vi "Init Msg Output.vi"() -> (2 "Msg Output":refnum<class "Msg Output.lvclass">)   [LabVIEW 2020, in "jettl.lvlib" / "Stop jettl Msg.lvlib" / "Stop Msg Output.lvlib"]
uses:
  Stop Msg Output.lvlib
  Msg Output/Msg Output.lvclass
  Stop Msg Output/Stop Msg Output.lvclass
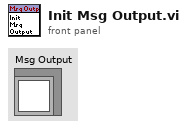
[diagram p1: front panel]
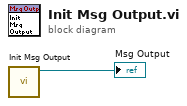
[diagram p0: block diagram]
diagram:
  n1 = call "Init Msg Output.vi"() -> ("Stop Msg Output out"=→"Msg Output":refnum<class "Stop Msg Output.lvclass">)  [unwired: 11 in]
